vi "Laser Initialization.vi"(3 "Serial Num":i32) -> (0 "error out":errorcluster, 1 "reference out":refnum<k7>)   [LabVIEW 2014]
panel:
  in  "APTLaser":refnum<k7>(container)
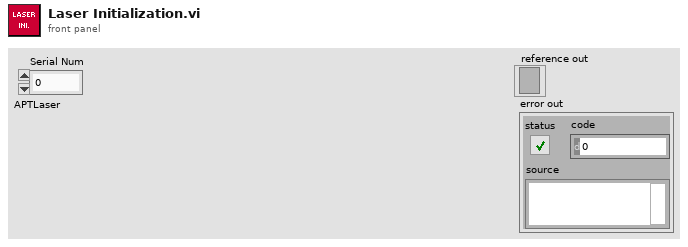
[diagram p1: front panel]
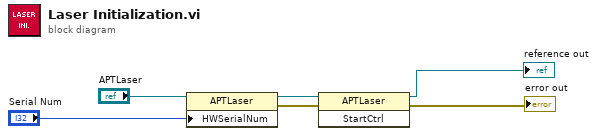
[diagram p0: block diagram]
diagram:
  n1 = property class="APTLaser"(reference="APTLaser", "HWSerialNum"="Serial Num") -> (reference out=w5:refnum<k7>, error out=w4:errorcluster)  [unwired: 1 in]
  n2 = invoke class="APTLaser" method="StartCtrl"(reference=w5, error in=w4) -> (reference out=→"reference out":refnum<k7>, error out=→"error out":errorcluster)  [unwired: 1 in, 1 out]
